vi "DAQmx Create Channel (CI-Two Edge Separation).vi"(0 "task in":refnum<k21>, 1 "maximum value":dbl=1.0 format="%0.6f", 2 "minimum value":dbl=1e-06 format="%0.6f", 5 "counter":tag, 7 "name to assign":string, 9 "units":i32(ring)=10364 items=["Seconds"=10364, "Ticks"=10304, "From Custom Scale"=10065], 11 "error in":errorcluster, 12 "custom scale name":tag, 13 "first edge":i32(ring)=10280 items=["Rising"=10280, "Falling"=10171], 14 "second edge":i32(ring)=10171 items=["Rising"=10280, "Falling"=10171]) -> (4 "task out":refnum<k21>, 15 "error out":errorcluster)   [LabVIEW 2011]
doc: "Creates a channel that measures the amount of time between the rising or falling edge of one digital signal and the rising or falling edge of another digital signal. You can create only one counter input channel at a time with this VI because a task can include only one counter input channel. To read from multiple counters simultaneously, use a separate task for each counter. Connect the input signals to the default input terminals of the counter unless you select different input terminals."
uses:
  C:/Program Files/National Instruments/LabVIEW 2011/resource/objmgr/daqmx.rc
panel:
  # "input limits"
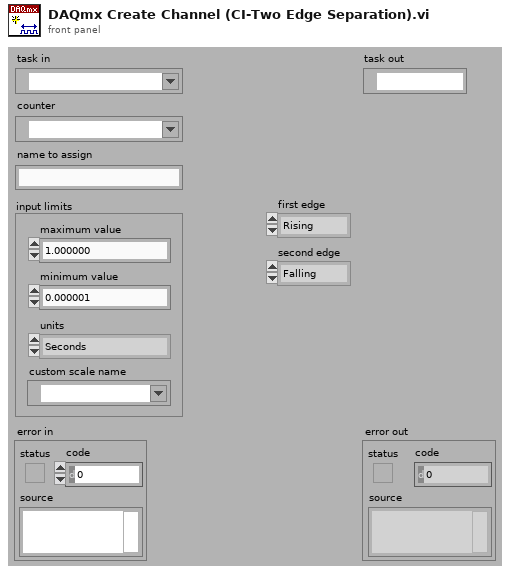
[diagram p1: front panel]
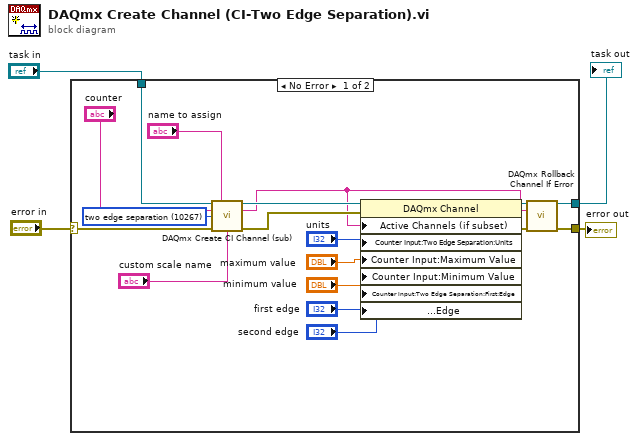
[diagram p0: block diagram]
diagram:
  n1 = case shown="No Error" "error in" {
    selector: "error in" -> [w21 w23]
    tunnel: "task in" -> [w22 w24]
    tunnel: [w12 w24] -> w2
    tunnel: [w10 w23] -> w1
    frame No Error {
      w5 = 10267 items=["count events"=10125, "frequency"=10179, "period"=10256, "pulse width"=10359, "semi period"=10289, "two edge separation"=10267, "angular encoder"=10360, "linear encoder"=0] ("measurement type")
      n2 = call "DAQmx Create CI Channel (sub).vi"("task in"=w22, "virtual channel name"="name to assign", "physical channel name"="counter", "measurement type"=w5, "error in"=w21, "custom scale"="custom scale name") -> ("task out"=w13:refnum<k21>, "channel names"=w8:string, "error out"=w19:errorcluster)  [unwired: 7 out]
      n3 = property class="DAQmx Channel"(reference=w13, error in=w19, "Active Channels (if subset)"=w8, "Counter Input:Two Edge Separation:Units"="units", "Counter Input:Maximum Value"="maximum value", "Counter Input:Minimum Value"="minimum value", "Counter Input:Two Edge Separation:First:Edge"="first edge", "Counter Input:Two Edge Separation:Second:Edge"="second edge") -> (reference out=w11:refnum<k21>, error out=w9:errorcluster)
      n4 = call "DAQmx Rollback Channel If Error.vi"("task in"=w11, "channel names"=w8, "error in"=w9) -> ("task out"=w12:refnum<k21>, "error out"=w10:errorcluster)  [unwired: 11 out]
    }
    frame Error {
    }
  }
  "error out" <- w1
  "task out" <- w2
